vi "室内外单幅图像-图片保存.vi"(9 "数据输入界限:最大值":dbl, 10 "路径":path) -> ()   [LabVIEW 2018]
panel:
  out "视频帧数":u32
  in  "下一步":bool
  in  "确定保存":bool
  out "Image":T1(plugin-control)
  in  "选择需要保存的帧数":u32=1 min=1 max=25
  # "图片保存"
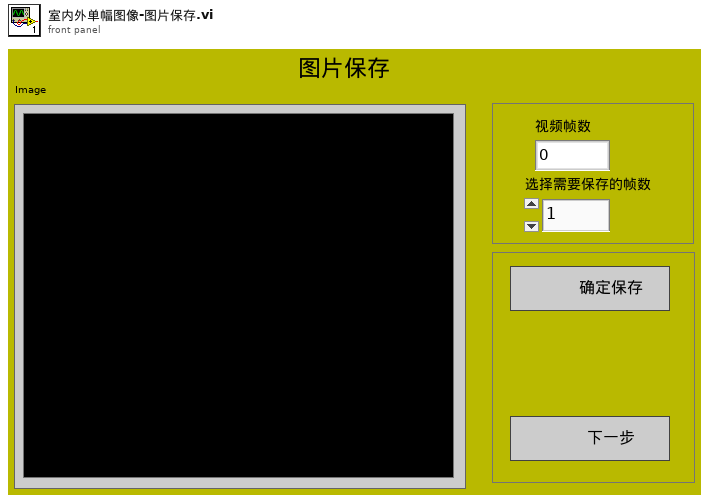
[diagram p1: front panel]
types:
  T1 = typedef "IMAQ Image.ctl" = refnum<image>
  T2 = enum8{"Enabled", "Disabled", "Disabled and Grayed Out"}
  T3 = typedef "Image Type" = u32
  T4 = typedef "IMAQ AVI2 Refnum.ctl" = refnum<k20>
  T5 = enum32{"Invalid", "Standard", "Closed", "Hidden", "Minimized", "Maximized"}
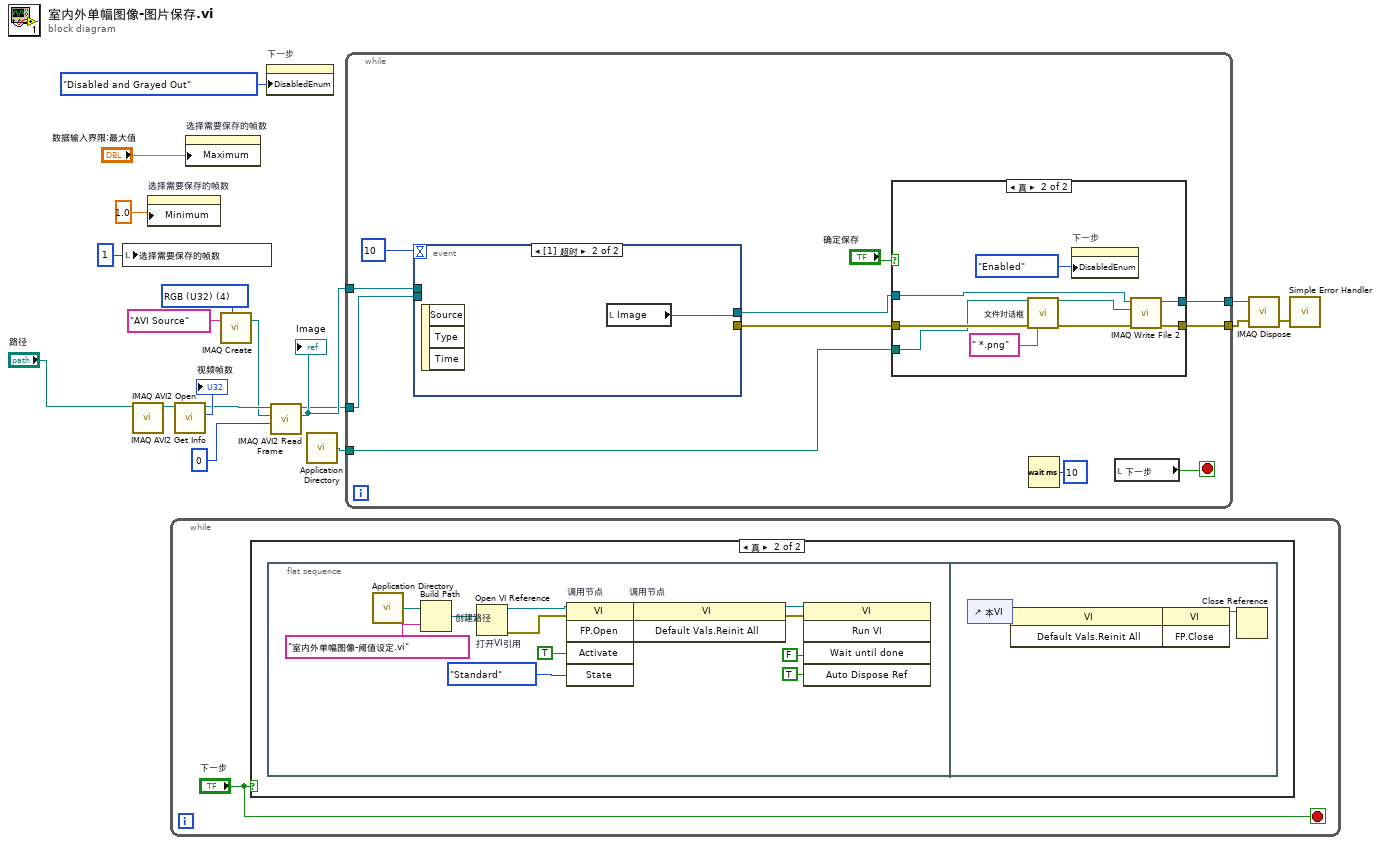
[diagram p0: block diagram]
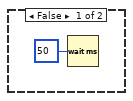
[diagram p2: hidden frame]
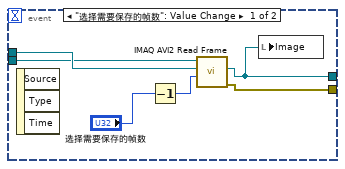
[diagram p3: hidden frame]
diagram:
  w15 = T3 4 items=["Grayscale (U8)", "Grayscale (I16)", "Grayscale (SGL)", "Complex (CSG)", "RGB (U32)", "HSL (U32)", "RGB (U64)", "Grayscale (U16)"] ("Image Type")
  n1 = local write "选择需要保存的帧数"(u32 1 ("选择需要保存的帧数")) -> ()
  n2 = call "IMAQ AVI2 Open"("AVI File Path"="路径") -> ("AVI Refnum"=w7:T4)  [unwired: 2 in, 8 out]
  n3 = property on="选择需要保存的帧数" class="DigNum (严格)"("Minimum"=1.0 ("数据输入界限:最小值")) -> ()  [unwired: 2 in, 2 out]
  n4 = while {
    stop <- "下一步" stop-if-true
    n5 = case shown="真" "下一步" {
      frame False {
        n6 = Wait (ms)(milliseconds to wait=u32 50 ("等待时间（毫秒）")) -> ()  [unwired: 1 out]
      }
      frame True {
        n7 = flat-sequence {
          frame #0 {
            n8 = call <vilib>:"Application Directory.vi"() -> ("Application Directory"=w21:path)
            n9 = Build Path "创建路径"(base path=w21, name or relative path="室内外单幅图像-阈值设定.vi" ("名称或相对路径")) -> (appended path=w31:path)
            n10 = Open VI Reference "打开VI引用"(vi path=w31) -> (vi reference=w30:refnum<vi>, error out=w29:errorcluster)  [unwired: 5 in]
            n11 = invoke on="调用节点" class="VI" method="FP.Open"(reference=w30, error in=w29, "Activate"=TRUE ("激活？"), "State"=T5."Standard" ("状态")) -> (reference out=w28:refnum<vi>, error out=w27:errorcluster)  [unwired: 1 in, 3 out]
            n12 = invoke on="调用节点" class="VI" method="Default Vals.Reinit All"(reference=w28, error in=w27) -> (reference out=w24:refnum<vi>, error out=w25:errorcluster)  [unwired: 1 in, 1 out]
            n13 = invoke class="VI" method="Run VI"(reference=w24, error in=w25, "Wait until done"=FALSE ("结束前等待"), "Auto Dispose Ref"=TRUE ("自动销毁引用")) -> ()  [unwired: 1 in, 5 out]
          }
          frame #1 {
            n14 = control-ref of="本VI"() -> (w36:refnum<vi>)
            n15 = invoke class="VI" method="Default Vals.Reinit All"(reference=w36) -> (reference out=w35:refnum<vi>)  [unwired: 2 in, 2 out]
            n16 = invoke class="VI" method="FP.Close"(reference=w35) -> (reference out=w34:refnum<vi>)  [unwired: 2 in, 2 out]
            n17 = Close Reference(reference=w34) -> ()  [unwired: 1 in, 1 out]
          }
        }
      }
    }
  }
  n18 = call "IMAQ AVI2 Get Info"("AVI Refnum"=w7) -> ("Number of Frames"=→"视频帧数":u32, "AVI Refnum (duplicate)"=w6:T4)  [unwired: 1 in, 8 out]
  n19 = property on="选择需要保存的帧数" class="DigNum (严格)"("Maximum"="数据输入界限:最大值") -> ()  [unwired: 2 in, 2 out]
  n20 = call "IMAQ Create"("Image Name"="AVI Source", "Image Type"=w15) -> ("New Image"=w3:T1)  [unwired: 2 in, 2 out]
  n21 = property on="下一步" class="Bool (严格)"("DisabledEnum"=T2."Disabled and Grayed Out" ("禁用")) -> ()  [unwired: 2 in, 2 out]
  n22 = call "IMAQ AVI2 Read Frame"("Frame Number"=u32 0, "Image"=w3, "AVI Refnum"=w6) -> ("Image Out"=w2:T1, "AVI Refnum (duplicate)"=w1:T4)  [unwired: 1 in, 6 out]
  "Image" <- w2
  n23 = call <vilib>:"Application Directory.vi"() -> ("Application Directory"=w14:path)
  n24 = while {
    tunnel: [w46] -> w17
    tunnel: [w45] -> w16
    tunnel: w14 -> [w44]
    tunnel: w2 -> [w41]
    tunnel: w1 -> [w38]
    stop <- w42 stop-if-true
    n25 = event shown="[1] 超时" {
      selector: _ -> [_ _]
      dyn-events: _ -> [_ _]
      timeout: 10 -> [_ _]
      tunnel: w41 -> [w51 _]
      tunnel: [w48 w54] -> w40
      tunnel: [w50 _] -> w39
      tunnel: w38 -> [w49 _]
      event "选择需要保存的帧数": Value Change {
        n26 = event-data() -> ()  [unwired: 1 in, 3 out]
        n27 = Decrement(x="选择需要保存的帧数") -> (x-1=w52:u32)
        n28 = call "IMAQ AVI2 Read Frame"("Frame Number"=w52, "Image"=w51, "AVI Refnum"=w49) -> ("error out"=w50:errorcluster, "Image Out"=w48:T1)  [unwired: 1 in, 6 out]
        n29 = local write "Image"(w48) -> ()
      }
      event Timeout {
        n30 = event-data() -> ()  [unwired: 1 in, 3 out]
        n31 = local read "Image"() -> (w54:T1)
      }
    }
    n32 = case shown="真" "确定保存" {
      tunnel: w40 -> [w56 w58]
      tunnel: [w56 w65] -> w46
      tunnel: w39 -> [w55 w62]
      tunnel: [w55 w64] -> w45
      tunnel: w44 -> [_ w60]
      frame False {
      }
      frame True {
        n33 = call "文件对话框"("start path"=w60, "error in"=w62, "pattern (all files)"=" *.png") -> ("selected path"=w63:path, "error out"=w61:errorcluster)  [unwired: 9 in, 2 out]
        n34 = property on="下一步" class="Bool (严格)"("DisabledEnum"=T2."Enabled" ("禁用")) -> ()  [unwired: 2 in, 2 out]
        n35 = call-poly "IMAQ Write File 2"("error in (no error)"=w61, "File Path"=w63, "Image"=w58) -> ("error out"=w64:errorcluster, "Image Out (duplicate)"=w65:T1)  [unwired: 7 in]
      }
    }
    n36 = Wait (ms)(milliseconds to wait=u32 10 ("等待时间（毫秒）")) -> ()  [unwired: 1 out]
    n37 = local read "下一步"() -> (w42:bool)
  }
  n38 = call "IMAQ Dispose"("Image"=w17, "error in (no error)"=w16) -> ("error out"=w12:errorcluster)  [unwired: 4 in]
  n39 = call <vilib>:"Simple Error Handler.vi"("error in (no error)"=w12) -> ()  [unwired: 4 in, 5 out]
